vi "LSX Connect Simple.vi"(6 "bAShowProt":i32, 7 "lABaudRate":i32, 8 "error in (no error)":errorcluster, 9 "pcAComName":string, 10 "lAnInterfaceType":i32, 11 "lLSID":i32) -> (0 "error out":errorcluster, 1 "pcAComName out":string, 3 "function return":i32)   [LabVIEW 2016, in "Tango_DLL.lvlib"]
doc: "TANGOAPI int TANGOCALL LSX_ConnectSimple (int lLSID, int lAnInterfaceType, char *pcAComName, int lABaudRate, BOOL bAShowProt);"
uses:
  Tango_DLL.lvlib
  Tango_DLL.dll
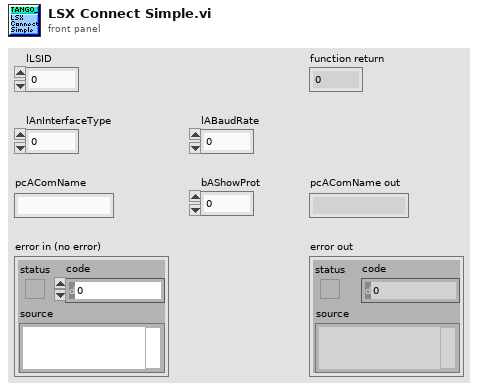
[diagram p1: front panel]
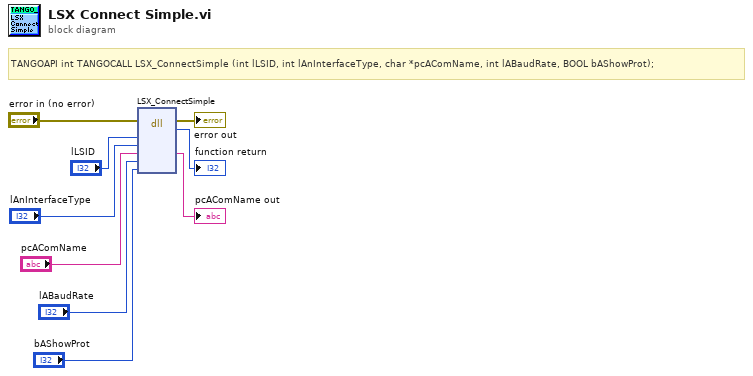
[diagram p0: block diagram]
diagram:
  # "TANGOAPI int TANGOCALL LSX_ConnectSimple (int lLSID, int lAnInterfaceType, char *pcAComName, int lABaudRate, BOOL bAShowProt);"
  n1 = dll-call lib="C:/Users/4PiSMS/Documents/Microscope Control/2016/Device Library/Stages/Marzhauser/SCAN IM 120 x 80/Tango DLL VIs/Tango_DLL.*" fn="LSX_ConnectSimple"(error in="error in (no error)", "lLSID"="lLSID", "lAnInterfaceType"="lAnInterfaceType", "pcAComName"="pcAComName", "lABaudRate"="lABaudRate", "bAShowProt"="bAShowProt") -> (error out=→"error out":errorcluster, →"function return":i32, "pcAComName"=→"pcAComName out":string)  [unwired: 6 in, 1 out]
